vi "Configure Channel Display.vi"(5 "Channel 2 Display With Ratio (0: None)":u16(ring) items=["None", "Aux In 3", "Aux In 4"], 7 "Channel 2 Display  (0: Y)":u16(ring) items=["Y", "Theta", "Y Noise", "Aux In 3", "Aux In 4"], 8 "error in (no error)":errorcluster, 9 "Channel 1 Display With Ratio (0: None)":u16(ring) items=["None", "Aux In 1", "Aux In 2"], 10 "Channel 1 Display (0: X)":u16(ring) items=["X", "R", "X Noise", "Aux In 1", "Aux In 2"], 11 "VISA resource name":refnum<visa-resource-name>) -> (0 "error out":errorcluster, 3 "VISA resource name out":refnum<visa-resource-name>)   [LabVIEW 2012, in "Stanford Research 830.lvlib"]
doc: "Configures the channel display of the instrument.\n\n<B>Note:</B>\n\nThe display will affect the value of the channel output."
uses:
  Stanford Research 830.lvlib
panel:
  # "Channel 1"
  # "Channel 2"
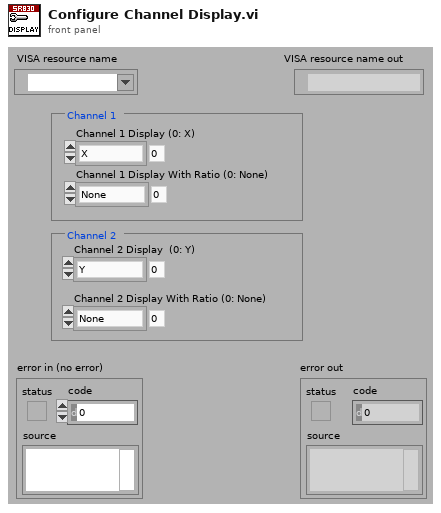
[diagram p1: front panel]
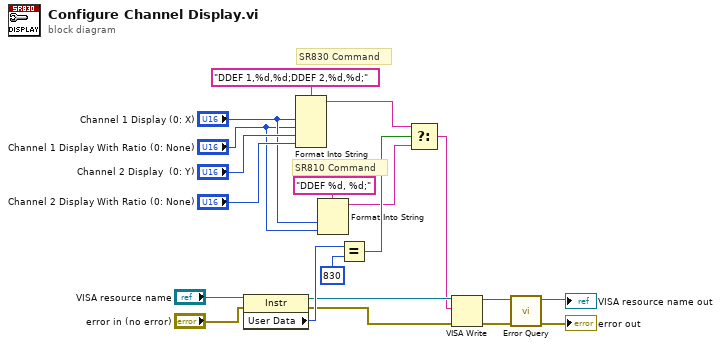
[diagram p0: block diagram]
diagram:
  # "SR810 Command"
  # "SR830 Command"
  n1 = property class="Instr"(reference="VISA resource name", error in="error in (no error)") -> (reference out=w9:refnum<visa-resource-name>, error out=w8:errorcluster, "User Data"=w13:u32)
  n2 = Format Into String(format string="DDEF 1,%d,%d;DDEF 2,%d,%d;", "Channel 1 Display (0: X)", "Channel 1 Display With Ratio (0: None)", "Channel 2 Display  (0: Y)", "Channel 2 Display With Ratio (0: None)") -> (resulting string=w6:string)  [unwired: 2 in, 1 out]
  n3 = Format Into String(format string="DDEF %d, %d;" ("initial string"), "Channel 1 Display (0: X)", "Channel 1 Display With Ratio (0: None)") -> (resulting string=w2:string)  [unwired: 2 in, 1 out]
  n4 = Equal?(x=w13, y=u32 830) -> (x = y?=w7:bool)
  n5 = Select(t=w6, s=w7, f=w2) -> (s? t:f=w1:string)
  n6 = VISA Write(VISA resource name=w9, write buffer=w1, error in (no error)=w8) -> (VISA resource name out=w17:refnum<visa-resource-name>, error out=w16:errorcluster)  [unwired: 1 out]
  n7 = call "Error Query.vi"("error in (no error)"=w16, "VISA resource name"=w17) -> ("error out"=→"error out":errorcluster, "VISA resource name out"=→"VISA resource name out":refnum<visa-resource-name>)  [unwired: 7 in, 1 out]
